vi "ProcessFile.vi"(8 "error in (no error)":errorcluster, 10 "Startup Analysis Configuration":T1, 11 "data in":T6) -> (0 "error out":errorcluster, 3 "data out":T6)   [LabVIEW 2017, in "McsaStartupAnalysis.lvlib"]
uses:
  <vilib>/addons/InsightCM/Devices/Shared/Mcsa/McsaStartupAnalysis/McsaStartupAnalysis.lvlib
  <vilib>/addons/InsightCM/Devices/Shared/Common/FileFlow/controls/data_eventRef.ctl
  <vilib>/addons/InsightCM/Devices/Shared/Common/DataEvent/controls/EventReference.ctl
  <vilib>/addons/InsightCM/Devices/Shared/Common/DataEvent/controls/Event.ctl
  <vilib>/addons/InsightCM/MessageBus/Base/controls/DataEvent.ctl
  <vilib>/addons/InsightCM/MessageBus/Base/controls/KeyValuePair.ctl
  <vilib>/addons/InsightCM/Devices/Shared/Common/DataEvent/controls/DataSet.ctl
  <vilib>/addons/InsightCM/MessageBus/Base/controls/DataSetMetadata.ctl
  <vilib>/addons/InsightCM/MessageBus/Base/controls/TrendPoint.ctl
  <vilib>/addons/InsightCM/MessageBus/Base/controls/TrendAlarmUpdate.ctl
  <vilib>/addons/InsightCM/MessageBus/Base/controls/TrendAlarmTransition.ctl
  <vilib>/addons/PointValueMap/controls/PointMap.ctl
  <vilib>/addons/InsightCM/Devices/Shared/Mcsa/McsaStartupAnalysis/controls/Config.ctl
  <vilib>/addons/InsightCM/Devices/Shared/Mcsa/McsaStartupAnalysis/controls/Group.ctl
  <vilib>/addons/InsightCM/Devices/Shared/Mcsa/McsaStartupAnalysis/controls/ChannelForStartup.ctl
  <vilib>/addons/InsightCM/Devices/Shared/Mcsa/McsaStartupAnalysis/controls/StartupFeature.ctl
  <vilib>/addons/InsightCM/Devices/Shared/Mcsa/McsaStartupAnalysis/controls/MotorInfo.ctl
  <vilib>/addons/PointValueMap/PointValueMap.lvlib
  <vilib>/addons/InsightCM/Devices/Shared/Common/DataEvent/DataEvent.lvlib
  <vilib>/addons/InsightCM/Devices/Shared/Common/FileFlow/FileFlow.lvlib
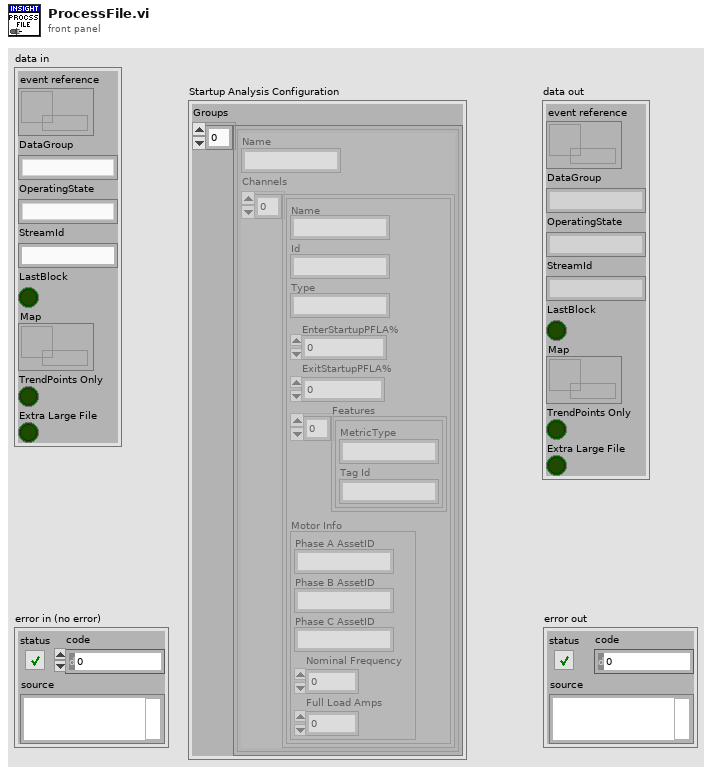
[diagram p1: front panel]
types:
  T1 = typedef "McsaStartupAnalysis.lvlib/Config.ctl" = cluster{"Groups":T2[]}
  T2 = typedef "McsaStartupAnalysis.lvlib/Group.ctl" = cluster{"Name":string, "Channels":T3[]}
  T3 = typedef "McsaStartupAnalysis.lvlib/ChannelForStartup.ctl" = cluster{"Name":string, "Id":string, "Type":string, "EnterStartupPFLA%":dbl, "ExitStartupPFLA%":dbl, "Features":T4[], "Motor Info":T5}
  T4 = typedef "McsaStartupAnalysis.lvlib/StartupFeature.ctl" = cluster{"MetricType":string, "Tag Id":string}
  T5 = typedef "McsaStartupAnalysis.lvlib/MotorInfo.ctl" = cluster{"Phase A AssetID":string, "Phase B AssetID":string, "Phase C AssetID":string, "Nominal Frequency":dbl, "Full Load Amps":dbl}
  T6 = typedef "FileFlow.lvlib/data_eventRef.ctl" = cluster{"event reference":T7, "DataGroup":string, "OperatingState":string, "StreamId":string, "LastBlock":bool, "Map":T8, "TrendPoints Only":bool, "Extra Large File":bool}
  T7 = typedef "DataEvent.lvlib/EventReference.ctl" = refnum<data-value>
  T8 = typedef "PointValueMap.lvlib/PointMap.ctl" = refnum<data-value>
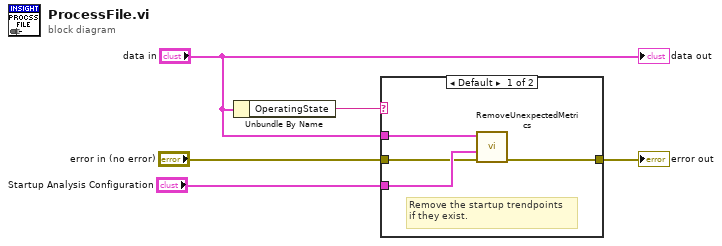
[diagram p0: block diagram]
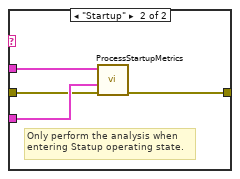
[diagram p2: hidden frame]
diagram:
  n1 = Unbundle By Name("data in") -> ("OperatingState"=w1:string)
  n2 = case shown="Default" w1 {
    tunnel: [w6 w13] -> w5
    tunnel: "error in (no error)" -> [w7 w11]
    tunnel: "Startup Analysis Configuration" -> [w9 w12]
    tunnel: "data in" -> [w8 w10]
    frame Default {
      # "Remove the startup trendpoints\nif they exist."
      n3 = call <vilib>:"RemoveUnexpectedMetrics.vi"("error in (no error)"=w7, "Startup Analysis Configuration"=w9, "data in"=w8) -> ("error out"=w6:errorcluster)  [unwired: 8 in]
    }
    frame "Startup" {
      # "Only perform the analysis when\nentering Statup operating state."
      n4 = call <vilib>:"ProcessStartupMetrics.vi"("error in (no error)"=w11, "Startup Analysis Configuration"=w12, "data in"=w10) -> ("error out"=w13:errorcluster)  [unwired: 8 in]
    }
  }
  "error out" <- w5
  "data out" <- "data in"
